vi "tearDown.vi"(8 "error in (no error)":errorcluster, 11 "reference in":refnum<class "UnitTestIntClass.lvclass">) -> (0 "error out":errorcluster, 3 "reference out":refnum<class "UnitTestIntClass.lvclass">)   [LabVIEW 2011, in "UnitTestIntClass.lvclass"]
doc: "tearDown runs after the test method has completed. Use this method to clean up any operations or references that were opened by setUp or the test method. Unit tests should be independent of other unit tests so this VI should ensure that the next test can run in a 'clean' test environment."
uses:
  UnitTestIntClass.lvclass
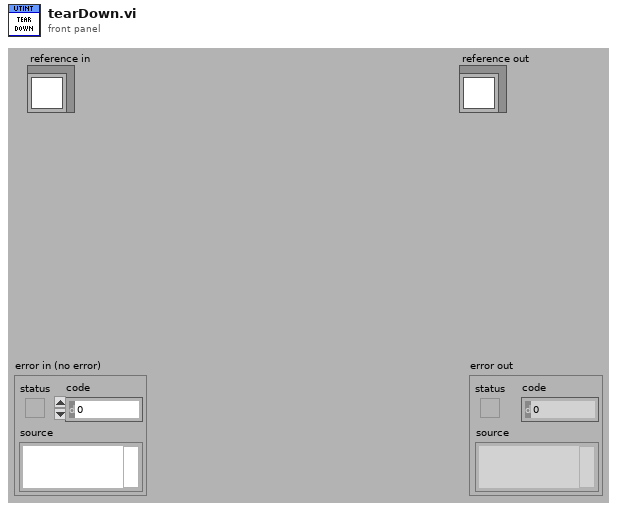
[diagram p1: front panel]
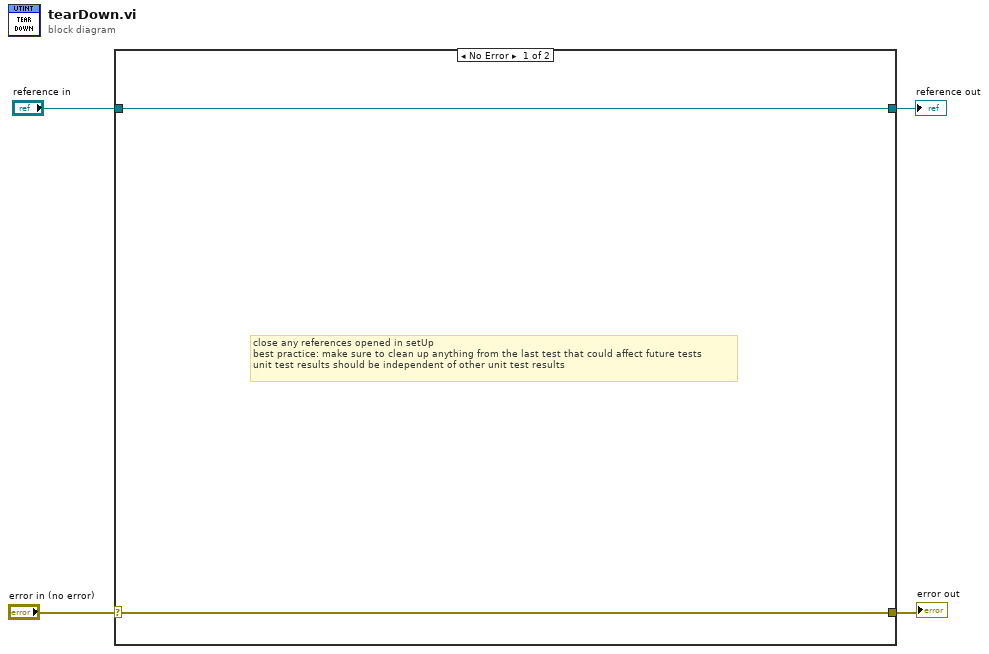
[diagram p0: block diagram]
diagram:
  n1 = case shown="No Error" "error in (no error)" {
    selector: "error in (no error)" -> [w5 w8]
    tunnel: [w5 w8] -> w3
    tunnel: [w6 w7] -> w1
    tunnel: "reference in" -> [w6 w7]
    frame No Error {
      # "close any references opened in setUp\nbest practice: make sure to clean up anything from the last test that could affect future tests\nunit test results should be independent of other unit test results"
    }
    frame Error {
    }
  }
  "error out" <- w3
  "reference out" <- w1
